vi "Update Dialog Box.vi"(8 "error in (no error)":errorcluster, 9 "Add EOL? (F)":bool, 10 "Text to add":string, 11 "Details Ref in":refnum<vi>) -> (0 "error out":errorcluster, 3 "Details Ref out":refnum<vi>)   [LabVIEW 2019, in "SEECD System Explorer.lvlib"]
uses:
  SEECD System Explorer.lvlib
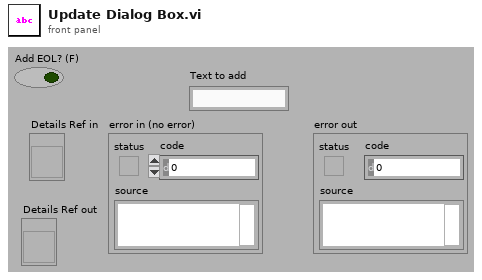
[diagram p1: front panel]
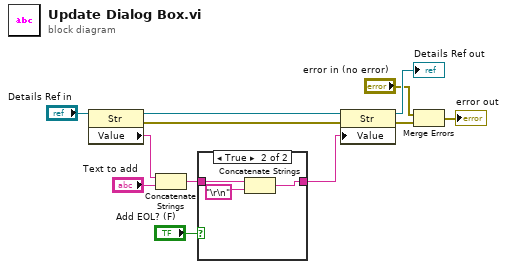
[diagram p0: block diagram]
diagram:
  n1 = property class="Str"(reference="Details Ref in") -> (reference out=w12:refnum<vi>, error out=w11:errorcluster, "Value"=w10:string)  [unwired: 1 in]
  n2 = Concatenate Strings(w10, "Text to add") -> (w3:string)
  n3 = case shown="True" "Add EOL? (F)" {
    tunnel: w3 -> [w13 w16]
    tunnel: [w13 w15] -> w1
    frame False {
    }
    frame True {
      n4 = Concatenate Strings(w16, "\r\n") -> (w15:string)
    }
  }
  n5 = property class="Str"(reference=w12, error in=w11, "Value"=w1) -> (reference out=→"Details Ref out":refnum<vi>, error out=w5:errorcluster)
  n6 = Merge Errors("error in (no error)", w5) -> (→"error out":errorcluster)
